vi "Remove Settings.vi"(8 "error in (no error)":errorcluster, 10 "Array":refnum<class "CommandSetting.lvclass">[](array[class]), 11 "WriteCommand in":refnum<class "WriteCommand.lvclass">) -> (0 "error out":errorcluster, 2 "Removed Count":u32, 3 "WriteCommand out":refnum<class "WriteCommand.lvclass">)   [LabVIEW 2023, in "HAF.lvlib" / "WriteCommand.lvclass"]
doc: "Removes the passed Command Settings from the collection currently held by the Command and returns a count of those actually removed."
uses:
  WriteCommand.lvclass
  WriteCommand.lvclass/WriteCommand.ctl
  CommandSetting/CommandSetting.lvclass
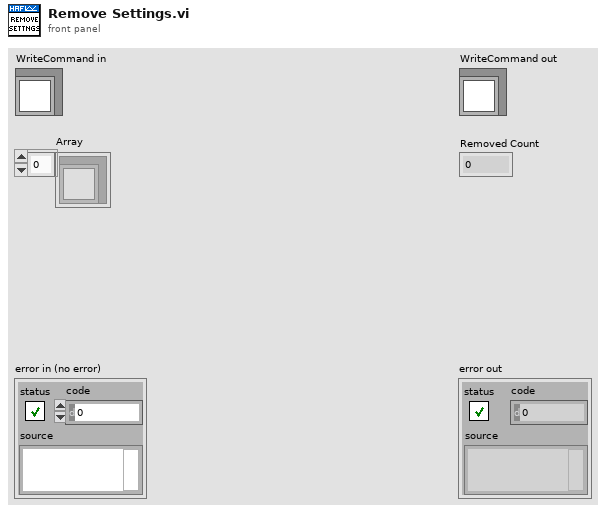
[diagram p1: front panel]
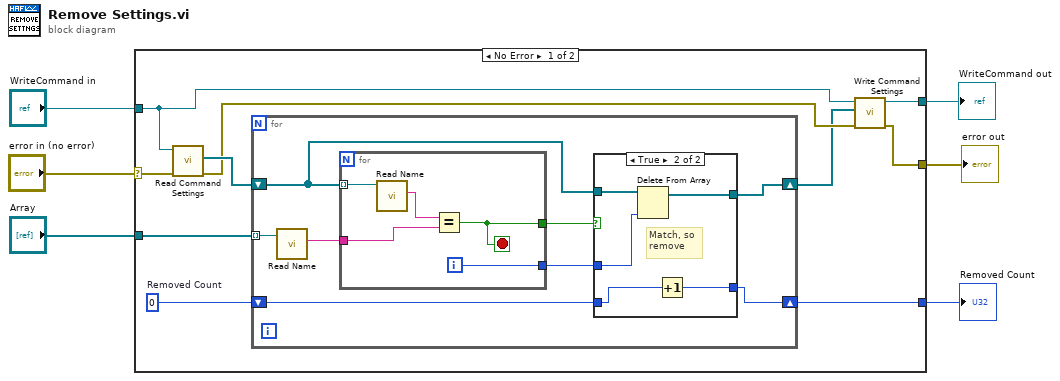
[diagram p0: block diagram]
diagram:
  n1 = case shown="No Error" "error in (no error)" {
    selector: "error in (no error)" -> [w16 w38]
    tunnel: [w8 w38] -> w2
    tunnel: [w9 w37] -> w3
    tunnel: "WriteCommand in" -> [w11 w37]
    tunnel: "Array" -> [w14 _]
    tunnel: [w7 _] -> w1
    frame No Error {
      w13 = u32 0  # Removed Count
      n2 = call-dynamic "Read Command Settings.vi"("error in (no error)"=w16, "WriteCommand in"=w11) -> ("error out"=w12:errorcluster, "Command Settings"=w15:refnum<class "CommandSetting.lvclass">[])  [unwired: 7 in, 1 out]
      n3 = for {
        shift-right: [w18] -> w10
        shift-left: w15 -> [w20]
        tunnel: w14 -> [w24] mode=indexing
        shift-right: [w17] -> w7
        shift-left: w13 -> [w19]
        n4 = call-dynamic "Read Name.vi"("Setting in"=w24) -> ("Name"=w23:string)  [unwired: 8 in, 2 out]
        n5 = for {
          tunnel: w20 -> [w36] mode=indexing
          tunnel: w23 -> [w34]
          tunnel: [w33] -> w22
          tunnel: [w32] -> w21
          i -> [w32]
          stop <- w33 stop-if-true
          n6 = call-dynamic "Read Name.vi"("Setting in"=w36) -> ("Name"=w35:string)  [unwired: 8 in, 2 out]
          n7 = Equal?(x=w35, y=w34) -> (x = y?=w33:bool)
        }
        n8 = case shown="True" w22 {
          tunnel: w21 -> [_ w30]
          tunnel: w20 -> [w26 w31]
          tunnel: w19 -> [w25 w29]
          tunnel: [w25 w28] -> w17
          tunnel: [w26 w27] -> w18
          frame False {
            # "No match so\nignore"
          }
          frame True {
            # "Match, so\nremove"
            n9 = Delete From Array(array=w31, index=w30) -> (array with subset deleted=w27:refnum<class "CommandSetting.lvclass">[])  [unwired: 1 in, 1 out]
            n10 = Increment(x=w29) -> (x+1=w28:u32)
          }
        }
      }
      n11 = call-dynamic "Write Command Settings.vi"("error in (no error)"=w12, "Command Settings"=w10, "WriteCommand in"=w11) -> ("error out"=w8:errorcluster, "WriteCommand out"=w9:refnum<class "WriteCommand.lvclass">)  [unwired: 7 in]
    }
    frame Error {
    }
  }
  "error out" <- w2
  "WriteCommand out" <- w3
  "Removed Count" <- w1
